vi "view -- cursor window logic.vi"() -> ()   [LabVIEW 2010]
uses:
  cursor winow.ctl
  <vilib>/event_ctls.llb/eventvkey.ctl
  cursor window action.ctl
panel:
  out "Char":i16
  out "VKey":T1
  in  "cursor window out":T2={"left"=2378.60310421286, "right "=2421.6740576496672, "center"=2421.6740576496672, "window"=2421.6740576496672, "cursors"=[], "relative"=0, "absolute"=0, "fixed vertical offset"=2421.6740576496672, "vertical offset"=2421.6740576496672, "skew"=2421.6740576496672, "default window frac"=2421.6740576496672, "kind"=enum."skewed", "skew.left"=2421.6740576496672, "skew.right"=2421.6740576496672, "Plot ref"=refnum, "wing order"=enum."back"}
  out "Plot: All":cluster{"all rows":dbl[], "all rows":dbl[]}[](graph)
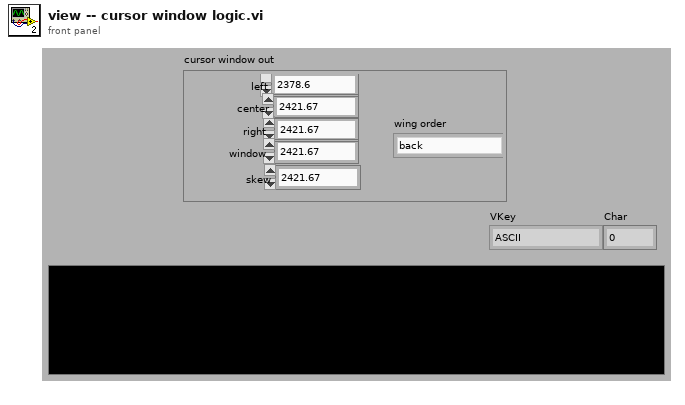
[diagram p1: front panel]
types:
  T1 = typedef "eventvkey.ctl" = enum16{"ASCII", "Enter", "Return", "Shift", "Ctrl", "Alt", "Cmd", "Opt", "Caps", "NumLock", "Clear", "Break", "Up", "Down", "Left", "Right", "Insert", "Delete", "Home", "End", "PageUp", "PageDown", "Escape", "Help", "Pause", "ScrollLock", "F1", "F2", "F3", "F4", "F5", "F6", "F7", "F8", "F9", "F10", "F11", "F12", "F13", "F14", "F15", "F16", "F17", "F18", "F19", "F20", "F21", "F22", "F23", "F24", "Play", "VolumeUp", "VolumeDown", "Mute", "Two Byte Char"}
  T2 = typedef "cursor winow.ctl" = cluster{"left":dbl, "right ":dbl, "center":dbl, "window":dbl, "cursors":i32[], "relative":i32, "absolute":i32, "fixed vertical offset":dbl, "vertical offset":dbl, "skew":dbl, "default window frac":dbl, "kind":enum16{"symmetric", "skewed", "fancy"}, "skew.left":dbl, "skew.right":dbl, "Plot ref":refnum<vi>, "wing order":enum16{"forw", "back"}}
  T3 = typedef "cursor window action.ctl" = enum16{"balance", "h. offset change", "cursor moves", "change center", "change window", "init", "check", "reset", "set y to middle", "idle", "-write all Y", "-write left.X", "-write center.X", "-write right.X", "-write all X", "-change center", "-change window", "-change skew", "-read cursor 2", "-read cursor 1", "-read cursor 0", "-read all cursors", "-reset", "-read plot scale", "-set y to middle", "-Q: center.Y is visible", "-Q: window is visible", "-parse center.Y", "-right left from center", "-left move", "-right move", "-set center.Y", "-empty", "-set cursors to default", "-check", "-write center.Y", "-copy cursor 1", "-copy cursor 0", "-copy cursor 2", "move right", "move left", "shrink", "broaden", "skew up", "skew down", "-write plot scale", "zoom X"}
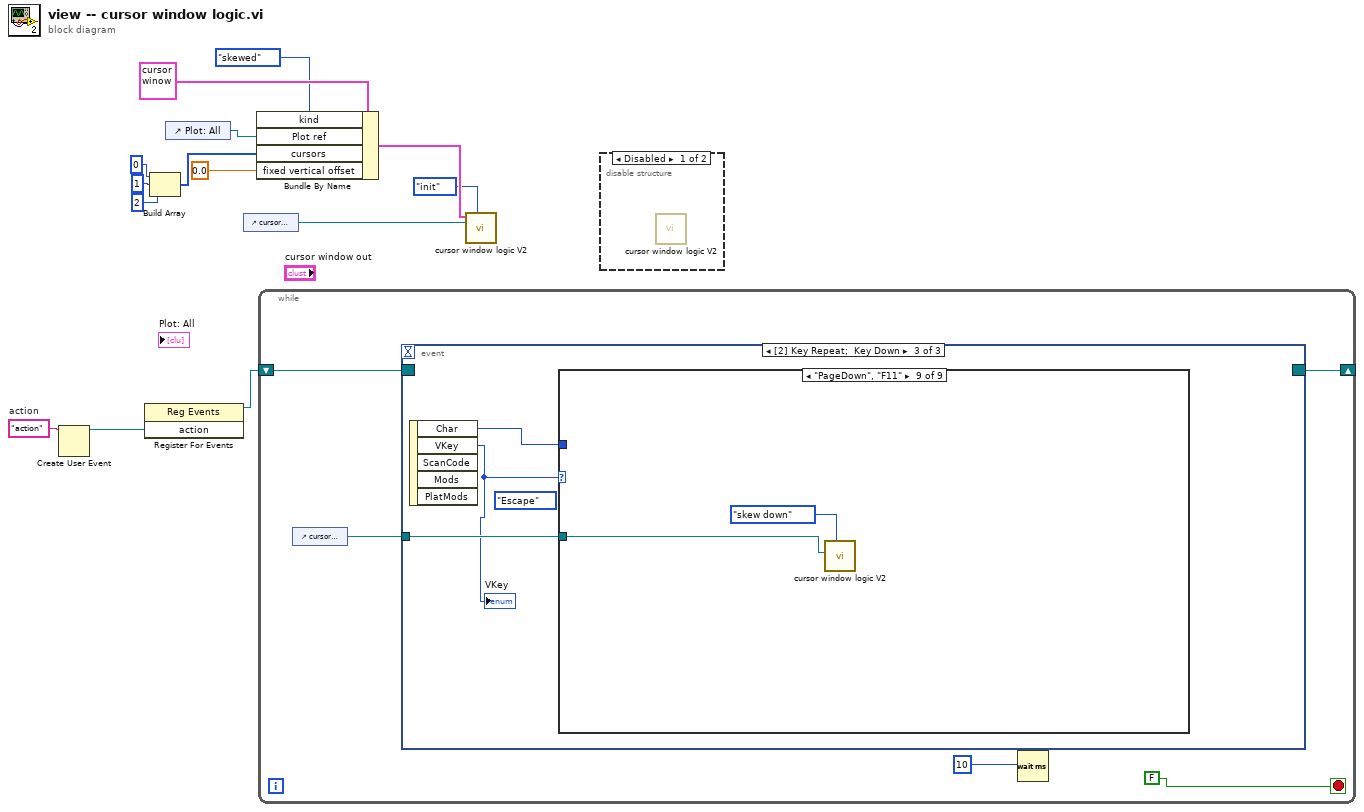
[diagram p0: block diagram]
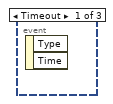
[diagram p3: hidden frame]
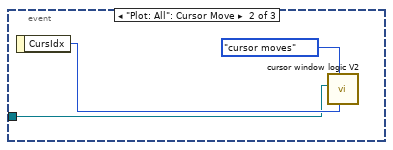
[diagram p4: hidden frame]
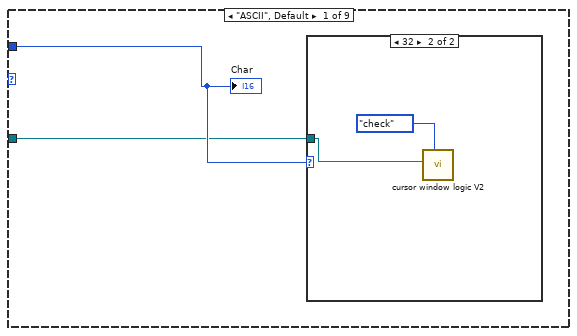
[diagram p5: hidden frame]
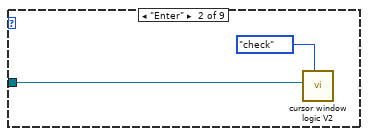
[diagram p7: hidden frame]
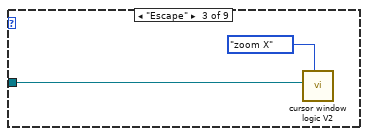
[diagram p8: hidden frame]
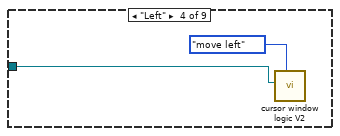
[diagram p9: hidden frame]
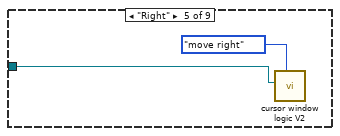
[diagram p10: hidden frame]
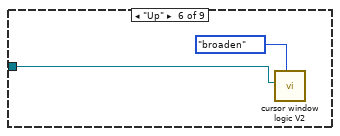
[diagram p11: hidden frame]
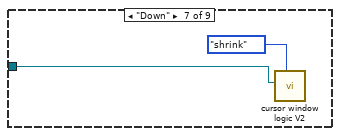
[diagram p12: hidden frame]
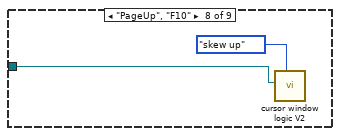
[diagram p13: hidden frame]
diagram:
  w3 = "action"  # action
  n1 = Create User Event(user event datatype=w3) -> (user event=w4:refnum<user-event>)  [unwired: 1 in, 1 out]
  n2 = register-events(w4) -> (reference out=w5:refnum<event-registration>)  [unwired: 2 in, 1 out]
  n3 = Build Array(0, 1, 2) -> (w14:i32[])
  n4 = control-ref of="Plot: All"() -> (w10:refnum<vi>)
  n5 = control-ref of="cursor window out"() -> (w7:refnum<vi>)
  n6 = Bundle By Name(cluster=T2 {"left"=2378.60310421286, "right "=2421.6740576496672, "center"=2421.6740576496672, "window"=2421.6740576496672, "cursors"=[], "relative"=0, "absolute"=0, "fixed vertical offset"=2421.6740576496672, "vertical offset"=2421.6740576496672, "skew"=2421.6740576496672, "default window frac"=2421.6740576496672, "kind"=enum."skewed", "skew.left"=2421.6740576496672, "skew.right"=2421.6740576496672, "Plot ref"=refnum, "wing order"=enum."back"} ("cursor window out"), "kind"=enum16{"symmetric", "skewed", "fancy"}."skewed", "Plot ref"=w10, "cursors"=w14, "fixed vertical offset"=0.0) -> (w9:T2)
  n7 = while {
    shift-right: [w15] -> _
    shift-left: w5 -> [w19]
    stop <- FALSE stop-if-true
    n8 = control-ref of="cursor window out"() -> (w18:refnum<vi>)
    n9 = event shown="[2] Key Repeat;  Key Down" {
      selector: w19 -> [_ _ _]
      dyn-events: [_ _ _] -> w15
      timeout: _ -> [_ _ _]
      tunnel: w18 -> [_ w20 w25]
      event Timeout {
        n10 = event-data() -> ()  [unwired: 1 in, 2 out]
      }
      event "Plot: All": Cursor Move {
        n11 = event-data() -> ("CursIdx"=w22:i32)  [unwired: 1 in]
        n12 = call "cursor window logic V2.vi"("CursIdx"=w22, "cursor window action"=cursor_window_action."cursor moves", "cursor window in"=w20) -> ()  [unwired: 7 in, 2 out]
      }
      event Key Repeat; Key Down {
        (unwired) eventvkey."Escape" ("VKey")
        n13 = event-data() -> ("Char"=w23:i16, "VKey"=w24:T1)  [unwired: 1 in, 3 out]
        "VKey" <- w24
        n14 = case shown="\"PageDown\", \"F11\"" w24 {
          tunnel: w25 -> [w26 w31 w33 w34 w36 w38 w40 w42 w44]
          tunnel: w23 -> [w27 _ _ _ _ _ _ _ _]
          frame "ASCII", Default {
            n15 = case shown="32" w27 {
              tunnel: w26 -> [_ w28]
              frame 0, Default {
              }
              frame 32 {
                n16 = call "cursor window logic V2.vi"("cursor window action"=cursor_window_action."check", "cursor window in"=w28) -> ()  [unwired: 8 in, 2 out]
              }
            }
            "Char" <- w27
          }
          frame "Enter" {
            n17 = call "cursor window logic V2.vi"("cursor window action"=cursor_window_action."check", "cursor window in"=w31) -> ()  [unwired: 8 in, 2 out]
          }
          frame "Escape" {
            n18 = call "cursor window logic V2.vi"("cursor window action"=cursor_window_action."zoom X", "cursor window in"=w33) -> ()  [unwired: 8 in, 2 out]
          }
          frame "Left" {
            n19 = call "cursor window logic V2.vi"("cursor window action"=cursor_window_action."move left", "cursor window in"=w34) -> ()  [unwired: 8 in, 2 out]
          }
          frame "Right" {
            n20 = call "cursor window logic V2.vi"("cursor window action"=cursor_window_action."move right", "cursor window in"=w36) -> ()  [unwired: 8 in, 2 out]
          }
          frame "Up" {
            n21 = call "cursor window logic V2.vi"("cursor window action"=cursor_window_action."broaden", "cursor window in"=w38) -> ()  [unwired: 8 in, 2 out]
          }
          frame "Down" {
            n22 = call "cursor window logic V2.vi"("cursor window action"=cursor_window_action."shrink", "cursor window in"=w40) -> ()  [unwired: 8 in, 2 out]
          }
          frame "PageUp", "F10" {
            n23 = call "cursor window logic V2.vi"("cursor window action"=cursor_window_action."skew up", "cursor window in"=w42) -> ()  [unwired: 8 in, 2 out]
          }
          frame "PageDown", "F11" {
            n24 = call "cursor window logic V2.vi"("cursor window action"=cursor_window_action."skew down", "cursor window in"=w44) -> ()  [unwired: 8 in, 2 out]
          }
        }
      }
    }
    n25 = Wait (ms)(milliseconds to wait=10) -> ()  [unwired: 1 out]
  }
  n26 = call "cursor window logic V2.vi"("cursor window action"=cursor_window_action."init", "cursor window in"=w7, "cursor window init"=w9) -> ()  [unwired: 7 in, 2 out]
  n27 = disable-structure shown="Disabled" {
    frame Disabled {
      n28 = call "cursor window logic V2.vi"() -> ()  [unwired: 10 in, 2 out]
    }
    frame Enabled {
    }
  }
